vi "TestExec.Configure Setup and Dialog.vi"(9 "Dialog":bool, 11 "Local Station Folder":path=path "C:/MTE/Test Executive/Config") -> (1 "Saved":bool, 2 "Data Out":variant, 3 "AppData out":refnum<class "Class.AppData.lvclass">)   [LabVIEW 2018]
uses:
  Common/Utils/TestExec/TestExec.WorkingDir.ctl
  <vilib>/KATE/Config/App Data/Class.AppData.lvclass
  Controls and Type Defs/TestExec.Config Dialog State.ctl
  <vilib>/Utility/config.llb/Write Key (String).vi
  <vilib>/KATE/Files/File Utils.lvlib
  <vilib>/Utility/config.llb/NI_LVConfig.lvlib
panel:
  out "Tab Control":enum32{"Inputs", "Data", "Outputs"}(tab)
  out "Exists_CfgFiles":bool[](array[boolean])
  out "Exists_ModeCfg":bool
  in  "Sequence":cluster{"Default":string}={"Default"="Undefined"}
  in  "Factory":cluster{"Location":string}={"Location"="Undefined"}
  in  "Route Check Enable":bool
  in  "Facility":cluster{"Name":string, "Location":string}={"Name"="Undefined", "Location"="Undefined"}
  in  "Station":T1={"Name"="Undefined", "PN"="Undefined", "SN"="Undefined", "Rev"="Undefined"}
  out "Additional Config Files":path[](array[path])
  in  "Mode Config File":path
  out "Local Station Config File":path=path "C:/MTE/Data/Eyetube Calibration/Capture"
  in  "Save":bool
  in  "Cancel":bool
  in  "Data Folders":T2[](array[typedef])=[{"Name"="ResultsLocalDir", "Path"=path "c:/MTE/Data/XML"}, {"Name"="ResultsExternalDir", "Path"=path "c:/MTE/Data/Results"}, {"Name"="DataArchiveDir", "Path"=path "c:/MTE/Data/Archive"}, {"Name"="DataSumArchiveDir", "Path"=path "c:/MTE/Data/ArchiveSum"}]
  # "Test Station Configuration"
  # "Name                                                                                                         Path"
  # "If this is empty, the default modes will be used."
  # "If a file is specified, it's contents will over write local settings."
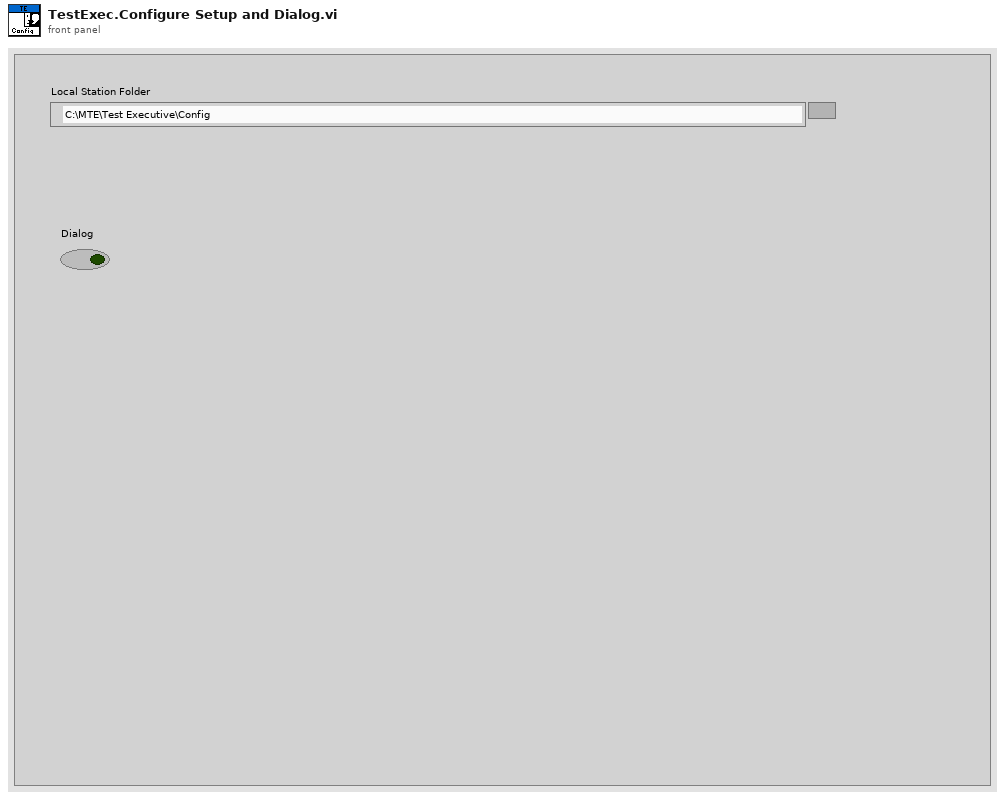
[diagram p1: front panel]
types:
  T1 = cluster{"Name":string, "PN":string, "SN":string, "Rev":string}
  T2 = typedef "TestExec.WorkingDir.ctl" = cluster{"Name":string, "Path":path}
  T3 = typedef "TestExec.Config Dialog State.ctl" = enum16{"Init", "Set Defaults", "Load Config", "Initialize Config", "Initialize Output", "Dialog", "Save", "Update Output", "Done"}
  T4 = enum32{"Invalid", "Standard", "Closed", "Hidden", "Minimized", "Maximized"}
  T5 = cluster{"Local Station Folder":path, "LocalCfgFile":path, "State":T3, "Save":bool, "Config":refnum<class "Class.AppData.lvclass">}
  T6 = typedef "NI_LVConfig.lvlib/Config Data RefNum.ctl" = refnum<k1>
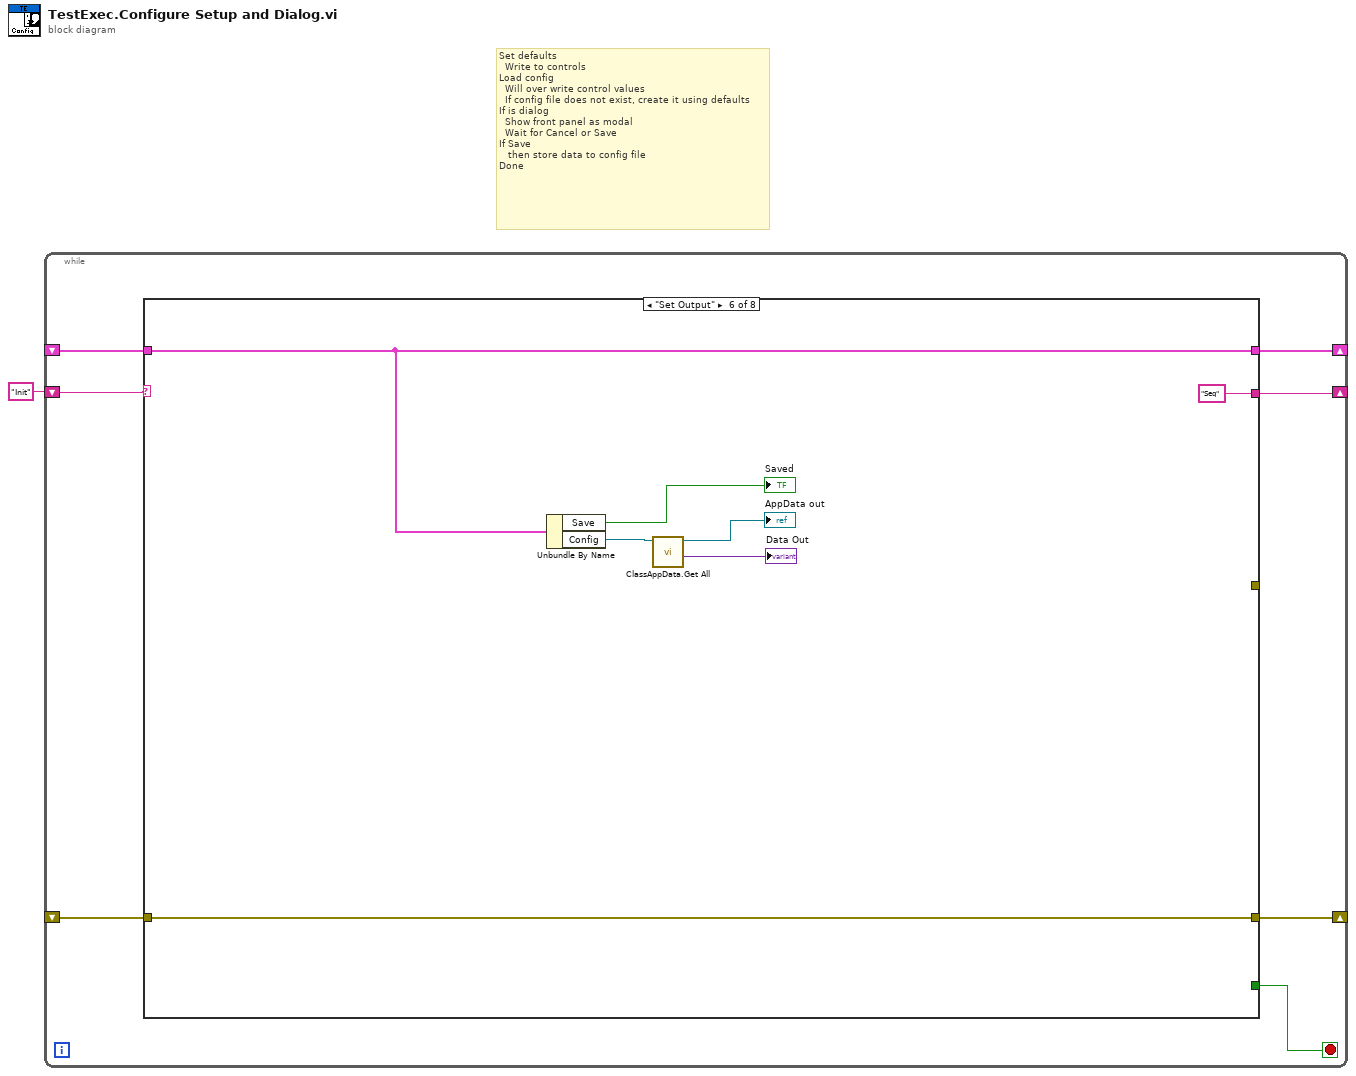
[diagram p0: block diagram]
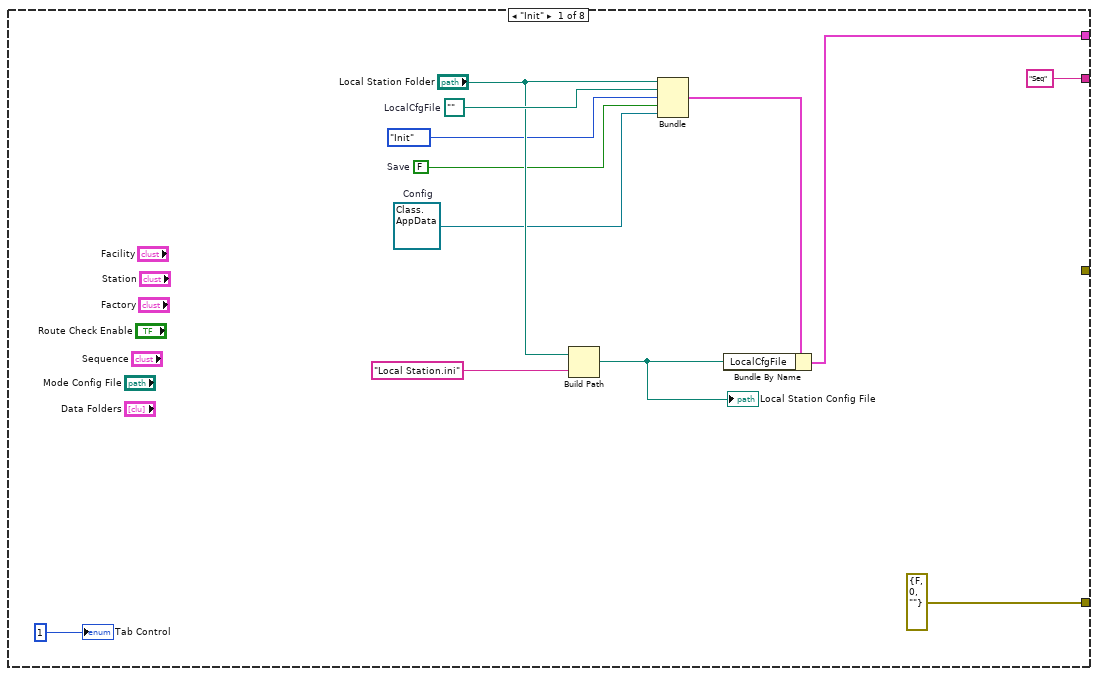
[diagram p2: hidden frame]
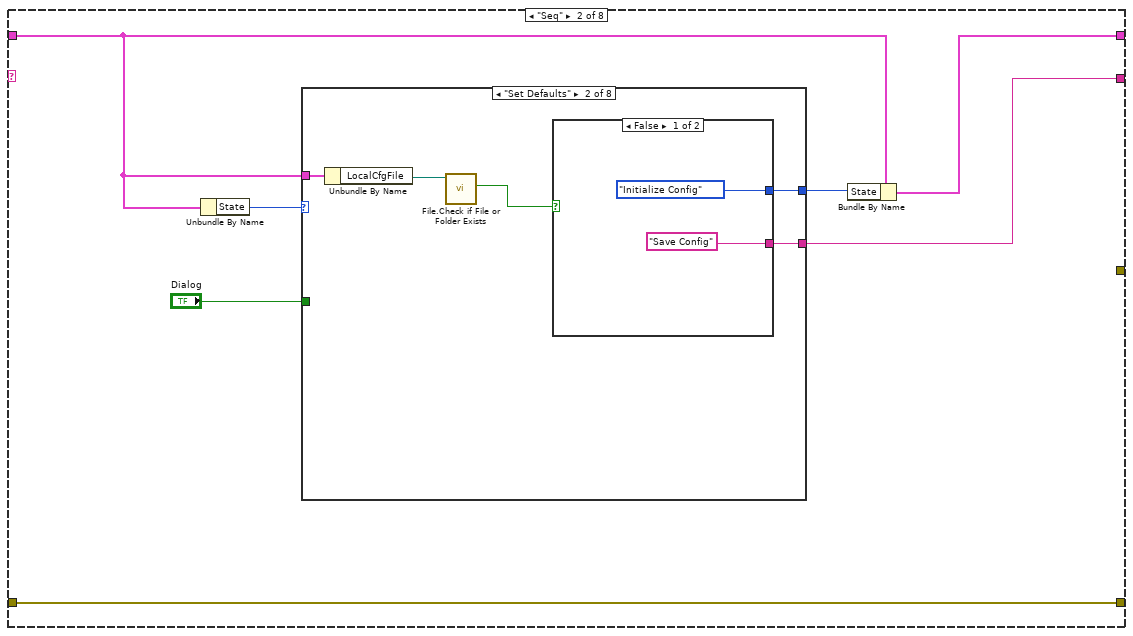
[diagram p3: hidden frame]
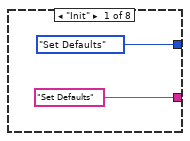
[diagram p4: hidden frame]
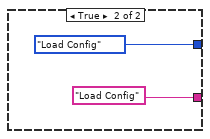
[diagram p5: hidden frame]
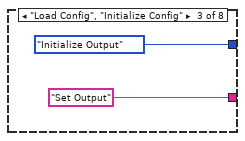
[diagram p6: hidden frame]
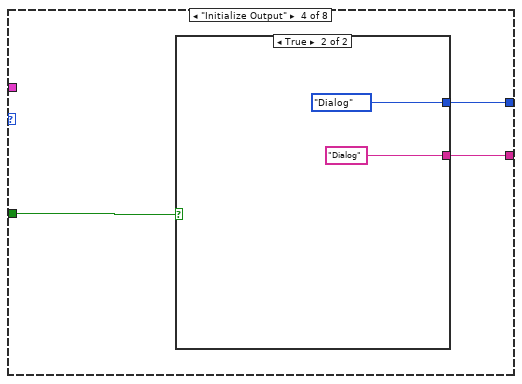
[diagram p7: hidden frame]
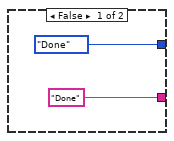
[diagram p8: hidden frame]
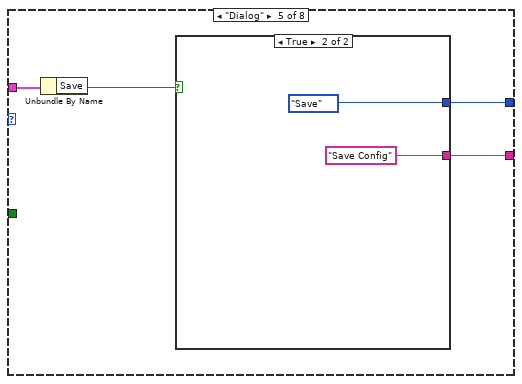
[diagram p9: hidden frame]
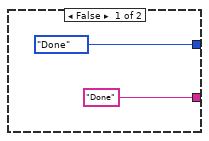
[diagram p10: hidden frame]
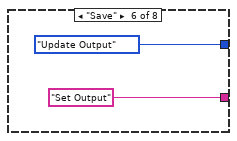
[diagram p11: hidden frame]
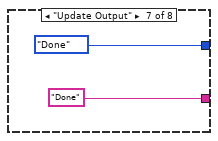
[diagram p12: hidden frame]
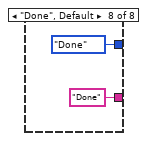
[diagram p13: hidden frame]
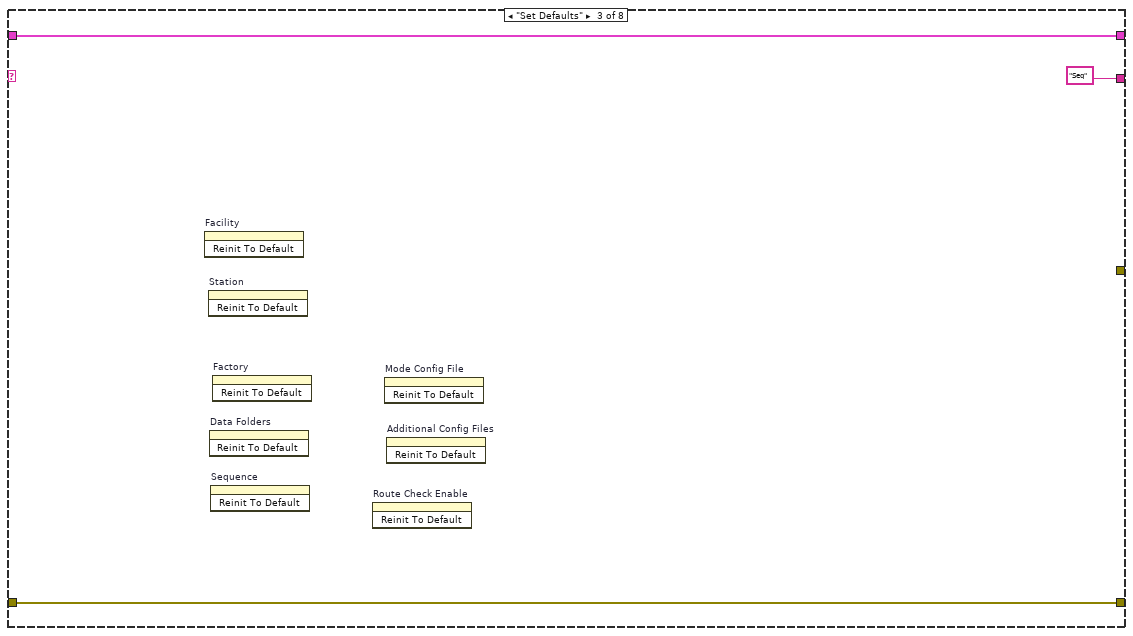
[diagram p14: hidden frame]
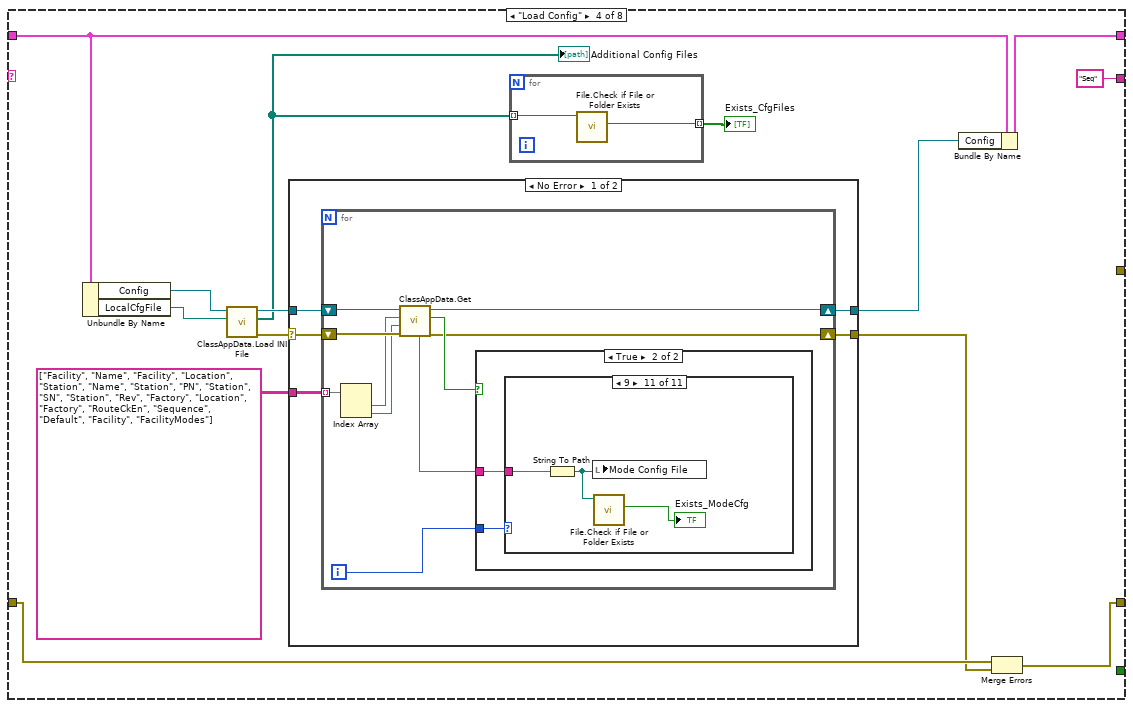
[diagram p15: hidden frame]
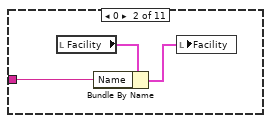
[diagram p18: hidden frame]
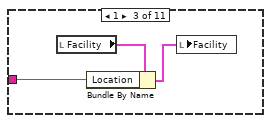
[diagram p19: hidden frame]
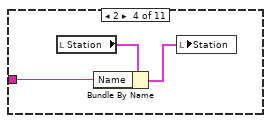
[diagram p20: hidden frame]
diagram:
  # "Set defaults\n  Write to controls\nLoad config\n  Will over write control values\n  If config file does not exist, create it using defaults\nIf is dialog\n  Show front panel as modal\n  Wait for Cancel or Save\nIf Save\n   then store data to config file\nDone"
  n1 = while {
    shift-right: [w6] -> _
    shift-left: _ -> [w8]
    shift-right: [w4] -> _
    shift-left: "Init" -> [w7]
    shift-right: [w2] -> _
    shift-left: _ -> [w3]
    stop <- w5 stop-if-true
    n2 = case shown="\"Set Output\"" w7 {
      tunnel: w8 -> [_ w25 w63 w77 w149 w189 w199 w219]
      tunnel: [w15 w24 w63 w76 w148 w189 w198 w219] -> w6
      tunnel: ["Seq" w22 "Seq" "Seq" "Seq" "Seq" w197 "Done"] -> w4
      tunnel: [_ _ _ _ _ _ _ TRUE] -> w5
      tunnel: [_ _ _ _ w139 _ _ _] -> _
      tunnel: w3 -> [_ w21 w62 w67 w138 w195 w196 w215]
      tunnel: [errorcluster {"status"=FALSE, "code"=0, "source"=""} ("error constant") w21 w62 w65 w135 w195 w196 w215] -> w2
      frame "Init" {
        w10 = refnum<class "Class.AppData.lvclass"> refnum  # Config
        w13 = FALSE  # Save
        w18 = path ""  # LocalCfgFile
        n3 = Build Path(base path="Local Station Folder", name or relative path="Local Station.ini") -> (appended path=w11:path)
        "Local Station Config File" <- w11
        n4 = Bundle("Local Station Folder"="Local Station Folder", "LocalCfgFile"=w18, "State"=TestExec.Config_Dialog_State."Init", "Save"=w13, "Config"=w10) -> (w16:T5)  [unwired: 1 in]
        n5 = Bundle By Name(cluster=w16, "LocalCfgFile"=w11) -> (w15:T5)
        "Tab Control" <- 1
      }
      frame "Seq" {
        n6 = Unbundle By Name(w25) -> ("State"=w27:T3)
        n7 = case shown="\"Set Defaults\"" w27 {
          tunnel: "Dialog" -> [_ _ _ w43 _ _ _ _]
          tunnel: w25 -> [_ w34 _ _ w49 _ _ _]
          tunnel: [TestExec.Config_Dialog_State."Set Defaults" ("State") w31 TestExec.Config_Dialog_State."Initialize Output" ("State") w42 w51 TestExec.Config_Dialog_State."Update Output" ("State") TestExec.Config_Dialog_State."Done" ("State") TestExec.Config_Dialog_State."Done" ("State")] -> w23
          tunnel: ["Set Defaults" w30 "Set Output" w41 w50 "Set Output" "Done" "Done"] -> w22
          frame "Init" {
          }
          frame "Set Defaults" {
            n8 = Unbundle By Name(w34) -> ("LocalCfgFile"=w33:path)
            n9 = call <vilib>:"File.Check if File or Folder Exists.vi"("Path"=w33) -> ("Exists"=w32:bool)  [unwired: 6 in, 4 out]
            n10 = case shown="False" w32 {
              tunnel: [TestExec.Config_Dialog_State."Initialize Config" ("State") TestExec.Config_Dialog_State."Load Config" ("State")] -> w31
              tunnel: ["Save Config" "Load Config"] -> w30
              frame False {
              }
              frame True {
              }
            }
          }
          frame "Load Config", "Initialize Config" {
          }
          frame "Initialize Output" {
            n11 = case shown="True" w43 {
              tunnel: [TestExec.Config_Dialog_State."Done" ("State") TestExec.Config_Dialog_State."Dialog" ("State")] -> w42
              tunnel: ["Done" "Dialog"] -> w41
              frame False {
              }
              frame True {
              }
            }
          }
          frame "Dialog" {
            n12 = Unbundle By Name(w49) -> ("Save"=w48:bool)
            n13 = case shown="True" w48 {
              tunnel: [TestExec.Config_Dialog_State."Done" ("State") TestExec.Config_Dialog_State."Save" ("State")] -> w51
              tunnel: ["Done" "Save Config"] -> w50
              frame False {
              }
              frame True {
              }
            }
          }
          frame "Save" {
          }
          frame "Update Output" {
          }
          frame "Done", Default {
          }
        }
        n14 = Bundle By Name(cluster=w25, "State"=w23) -> (w24:T5)
      }
      frame "Set Defaults" {
        n15 = invoke on="Facility" class="Clust (strict)" method="Reinit To Default"() -> ()  [unwired: 3 in, 3 out]
        n16 = invoke on="Station" class="Clust (strict)" method="Reinit To Default"() -> ()  [unwired: 3 in, 3 out]
        n17 = invoke on="Data Folders" class="Arr (strict)" method="Reinit To Default"() -> ()  [unwired: 3 in, 3 out]
        n18 = invoke on="Sequence" class="Clust (strict)" method="Reinit To Default"() -> ()  [unwired: 3 in, 3 out]
        n19 = invoke on="Factory" class="Clust (strict)" method="Reinit To Default"() -> ()  [unwired: 3 in, 3 out]
        n20 = invoke on="Route Check Enable" class="Bool (strict)" method="Reinit To Default"() -> ()  [unwired: 3 in, 3 out]
        n21 = invoke on="Mode Config File" class="Path" method="Reinit To Default"() -> ()  [unwired: 3 in, 3 out]
        n22 = invoke on="Additional Config Files" class="Arr (strict)" method="Reinit To Default"() -> ()  [unwired: 3 in, 3 out]
      }
      frame "Load Config" {
        n23 = Unbundle By Name(w77) -> ("Config"=w75:refnum<class "Class.AppData.lvclass">, "LocalCfgFile"=w74:path)
        n24 = call <vilib>:"ClassAppData.Load INI File.vi"("INI File"=w74, "Class - App Data in"=w75) -> ("error out"=w72:errorcluster, "Additional Cfg Files"=w68:path[], "Class - App Data out"=w73:refnum<class "Class.AppData.lvclass">)  [unwired: 7 in]
        "Additional Config Files" <- w68
        n25 = case shown="No Error" w72 {
          selector: w72 -> [w84 _]
          tunnel: w73 -> [w85 w132]
          tunnel: [w83 w132] -> w71
          tunnel: string[][] [["Facility", "Name"], ["Facility", "Location"], ["Station", "Name"], ["Station", "PN"], ["Station", "SN"], ["Station", "Rev"], ["Factory", "Location"], ["Factory", "RouteCkEn"], ["Sequence", "Default"], ["Facility", "FacilityModes"]] -> [w82 _]
          tunnel: [w81 _] -> w66
          frame No Error {
            n26 = for {
              shift-right: [w89] -> w83
              shift-left: w85 -> [w95]
              shift-right: [w88] -> w81
              shift-left: w84 -> [w94]
              tunnel: w82 -> [w93] mode=indexing
              i -> [w86]
              n27 = Index Array(array=w93) -> (element #1=w92:string, element #2=w91:string)  [unwired: 2 in]
              n28 = call <vilib>:"ClassAppData.Get.vi"("error in (no error)"=w94, "Name"=w91, "Section"=w92, "Class - App Data in"=w95) -> ("error out"=w88:errorcluster, "Found"=w90:bool, "Class - App Data out"=w89:refnum<class "Class.AppData.lvclass">, "String Data"=w87:string)  [unwired: 3 in, 1 out]
              n29 = case shown="True" w90 {
                tunnel: w87 -> [_ w96]
                tunnel: w86 -> [_ w97]
                frame False {
                  # "Skip"
                }
                frame True {
                  n30 = case shown="9" w97 {
                    tunnel: w96 -> [_ w98 w101 w104 w107 w110 w113 w116 w124 w126 w131]
                    frame Default {
                    }
                    frame 0 {
                      n31 = local read "Facility"() -> (w100:cluster{"Name":string, "Location":string})
                      n32 = Bundle By Name(cluster=w100, "Name"=w98) -> (w99:cluster{"Name":string, "Location":string})
                      n33 = local write "Facility"(w99) -> ()
                    }
                    frame 1 {
                      n34 = local read "Facility"() -> (w103:cluster{"Name":string, "Location":string})
                      n35 = Bundle By Name(cluster=w103, "Location"=w101) -> (w102:cluster{"Name":string, "Location":string})
                      n36 = local write "Facility"(w102) -> ()
                    }
                    frame 2 {
                      n37 = local read "Station"() -> (w106:T1)
                      n38 = Bundle By Name(cluster=w106, "Name"=w104) -> (w105:T1)
                      n39 = local write "Station"(w105) -> ()
                    }
                    frame 3 {
                      n40 = local read "Station"() -> (w109:T1)
                      n41 = Bundle By Name(cluster=w109, "PN"=w107) -> (w108:T1)
                      n42 = local write "Station"(w108) -> ()
                    }
                    frame 4 {
                      n43 = local read "Station"() -> (w112:T1)
                      n44 = Bundle By Name(cluster=w112, "SN"=w110) -> (w111:T1)
                      n45 = local write "Station"(w111) -> ()
                    }
                    frame 5 {
                      n46 = local read "Station"() -> (w115:T1)
                      n47 = Bundle By Name(cluster=w115, "Rev"=w113) -> (w114:T1)
                      n48 = local write "Station"(w114) -> ()
                    }
                    frame 6 {
                      n49 = local read "Factory"() -> (w118:cluster{"Location":string})
                      n50 = Bundle By Name(cluster=w118, "Location"=w116) -> (w117:cluster{"Location":string})
                      n51 = local write "Factory"(w117) -> ()
                    }
                    frame 7 {
                      n52 = To Upper Case(1:w124) -> (0:w125:string)
                      n53 = Equal?(x="1" ("y"), y=w124) -> (x = y?=w120:bool)
                      n54 = Equal?(x=w125, y="TRUE") -> (x = y?=w121:bool)
                      n55 = Or(x=w120, y=w121) -> (x .or. y?=w119:bool)
                      n56 = local write "Route Check Enable"(w119) -> ()
                    }
                    frame 8 {
                      n57 = local read "Sequence"() -> (w128:cluster{"Default":string})
                      n58 = Bundle By Name(cluster=w128, "Default"=w126) -> (w127:cluster{"Default":string})
                      n59 = local write "Sequence"(w127) -> ()
                    }
                    frame 9 {
                      n60 = String To Path(string=w131) -> (path=w130:path)
                      n61 = local write "Mode Config File"(w130) -> ()
                      n62 = call <vilib>:"File.Check if File or Folder Exists.vi"("Path"=w130) -> ("Exists"=→"Exists_ModeCfg":bool)  [unwired: 6 in, 4 out]
                    }
                  }
                }
              }
            }
          }
          frame Error {
          }
        }
        n63 = for {
          tunnel: w68 -> [w80] mode=indexing
          tunnel: [w79] -> w69 mode=indexing
          n64 = call <vilib>:"File.Check if File or Folder Exists.vi"("Path"=w80) -> ("Exists"=w79:bool)  [unwired: 6 in, 4 out]
        }
        "Exists_CfgFiles" <- w69
        n65 = Bundle By Name(cluster=w77, "Config"=w71) -> (w76:T5)
        n66 = Merge Errors(w67, w66) -> (w65:errorcluster)
      }
      frame "Save Config" {
        n67 = Unbundle By Name(w149) -> ("LocalCfgFile"=w143:path, "Config"=w145:refnum<class "Class.AppData.lvclass">)
        n68 = call <vilib>:"Open Config Data.vi"("create file if necessary (T)"=TRUE, "configuration file path"=w143) -> ("error out"=w134:errorcluster, "refnum"=w142:T6)  [unwired: 7 in, 1 out]
        n69 = for {
          shift-right: [w161] -> w147
          shift-left: w145 -> [w164]
          shift-right: [w160] -> w137
          shift-left: errorcluster {"status"=FALSE, "code"=0, "source"=""} ("error constant") -> [w163]
          tunnel: string[][] [["Facility", "Name"], ["Facility", "Location"], ["Station", "Name"], ["Station", "PN"], ["Station", "SN"], ["Station", "Rev"], ["Factory", "Location"], ["Factory", "RouteCkEn"], ["Sequence", "Default"], ["Facility", "FacilityModes"]] -> [w162] mode=indexing
          shift-right: [w151] -> w136
          shift-left: w134 -> [w156]
          shift-right: [w152] -> w140
          shift-left: w142 -> [w157]
          i -> [w159]
          n70 = Index Array(array=w162) -> (element #1=w154:string, element #2=w155:string)  [unwired: 2 in]
          n71 = case shown="9" w159 {
            tunnel: [_ w165 w167 w170 w172 w174 w176 w178 w179 w183 w186] -> w153
            frame Default {
            }
            frame 0 {
              n72 = local read "Facility"() -> (w166:cluster{"Name":string, "Location":string})
              n73 = Unbundle By Name(w166) -> ("Name"=w165:string)
            }
            frame 1 {
              n74 = local read "Facility"() -> (w168:cluster{"Name":string, "Location":string})
              n75 = Unbundle By Name(w168) -> ("Location"=w167:string)
            }
            frame 2 {
              n76 = local read "Station"() -> (w169:T1)
              n77 = Unbundle By Name(w169) -> ("Name"=w170:string)
            }
            frame 3 {
              n78 = local read "Station"() -> (w171:T1)
              n79 = Unbundle By Name(w171) -> ("PN"=w172:string)
            }
            frame 4 {
              n80 = local read "Station"() -> (w173:T1)
              n81 = Unbundle By Name(w173) -> ("SN"=w174:string)
            }
            frame 5 {
              n82 = local read "Station"() -> (w175:T1)
              n83 = Unbundle By Name(w175) -> ("Rev"=w176:string)
            }
            frame 6 {
              n84 = local read "Factory"() -> (w177:cluster{"Location":string})
              n85 = Unbundle By Name(w177) -> ("Location"=w178:string)
            }
            frame 7 {
              n86 = local read "Route Check Enable"() -> (w180:bool)
              n87 = Select(t="TRUE" ("y"), s=w180, f="FALSE" ("y")) -> (s? t:f=w179:string)
            }
            frame 8 {
              n88 = local read "Sequence"() -> (w184:cluster{"Default":string})
              n89 = Unbundle By Name(w184) -> ("Default"=w183:string)
            }
            frame 9 {
              n90 = local read "Mode Config File"() -> (w187:path)
              n91 = call <vilib>:"File.Check if File or Folder Exists.vi"("Path"=w187) -> ("Exists"=w188:bool, "Dup Path"=w185:path)  [unwired: 6 in, 3 out]
              n92 = Path To String(path=w185) -> (string=w186:string)
              n93 = local write "Exists_ModeCfg"(w188) -> ()
            }
          }
          n94 = To Variant(anything=w153) -> (Variant=w158:variant)
          n95 = call <vilib>:"ClassAppData.Set.vi"("Section"=w154, "error in (no error)"=w163, "Value"=w158, "Name"=w155, "Class - App Data in"=w164) -> ("error out"=w160:errorcluster, "Class - App Data out"=w161:refnum<class "Class.AppData.lvclass">)  [unwired: 4 in, 1 out]
          n96 = call-poly <vilib>:"Write Key.vi"("section"=w154, "error in (no error)"=w156, "value"=w153, "key"=w155, "refnum"=w157) -> ("error out"=w151:errorcluster, "refnum out"=w152:T6)  [unwired: 4 in, 1 out]
        }
        n97 = call <vilib>:"Close Config Data.vi"("error in (no error)"=w136, "write file if changed (T)"=TRUE, "refnum"=w140) -> ("error out"=w139:errorcluster)  [unwired: 7 in, 1 out]
        n98 = Bundle By Name(cluster=w149, "Config"=w147) -> (w148:T5)
        n99 = Merge Errors(w138, w137, w136) -> (w135:errorcluster)
      }
      frame "Set Output" {
        n100 = Unbundle By Name(w189) -> ("Save"=→"Saved":bool, "Config"=w191:refnum<class "Class.AppData.lvclass">)
        n101 = call <vilib>:"ClassAppData.Get All.vi"("Class - App Data in"=w191) -> ("Data Out"=→"Data Out":variant, "Class - App Data out"=→"AppData out":refnum<class "Class.AppData.lvclass">)  [unwired: 8 in, 1 out]
      }
      frame "Dialog" {
        n102 = control-ref of="This VI"() -> (w205:refnum<vi>)
        n103 = invoke class="VI" method="FP.Open"(reference=w205, "Activate"=TRUE ("Activate?"), "State"=T4."Standard") -> (reference out=w202:refnum<vi>, error out=w201:errorcluster)  [unwired: 2 in, 3 out]
        n104 = Close Reference(reference=w202, error in (no error)=w201) -> (error out=w200:errorcluster)
        n105 = while {
          tunnel: w200 -> [_]
          shift-right: [w207] -> w198
          shift-left: w199 -> [w208]
          tunnel: [w206] -> w197
          stop <- w209 stop-if-true
          n106 = event shown="[0] \"Cancel\", \"Save\": Value Change;  Panel Close" {
            selector: _ -> [_]
            dyn-events: _ -> [_]
            timeout: _ -> [_]
            tunnel: [TRUE] -> w209
            tunnel: w208 -> [w212]
            tunnel: [w211] -> w207
            tunnel: ["Seq"] -> w206
            event "Cancel", "Save": Value Change; Panel Close {
              n107 = event-data() -> ()  [unwired: 1 in, 3 out]
              n108 = Bundle By Name(cluster=w212, "Save"="Save") -> (w211:T5)
            }
          }
        }
      }
      frame "Done", Default {
        w217 = TRUE  # Normal(T)/Debug(F)
        n109 = local read "Dialog"() -> (w218:bool)
        n110 = And(x=w218, y=w217) -> (x .and. y?=w216:bool)
        n111 = case shown="True" w216 {
          tunnel: [_ w222] -> _
          frame False {
          }
          frame True {
            n112 = control-ref of="This VI"() -> (w225:refnum<vi>)
            n113 = invoke class="VI" method="FP.Close"(reference=w225) -> (reference out=w224:refnum<vi>, error out=w223:errorcluster)  [unwired: 2 in, 1 out]
            n114 = Close Reference(reference=w224, error in (no error)=w223) -> (error out=w222:errorcluster)
          }
        }
      }
    }
  }
